vi "JV SNAKE AND LADDERS.vi"() -> ()   [LabVIEW 2018]
panel:
  out "String":string="PLAYER ONE TURN"
  out "Boolean":bool
  out "?":bool
  out "PLAYER 2 position":dbl
  out "PLAYER 1 position":dbl
  out "String 2":string="PLAYER TWO TURN"
  out "VALUE YOU GOT":dbl
  in  "stop":bool
  in  "THROW":bool
  out "Numeric":dbl
  out "DICE":u16(ring)
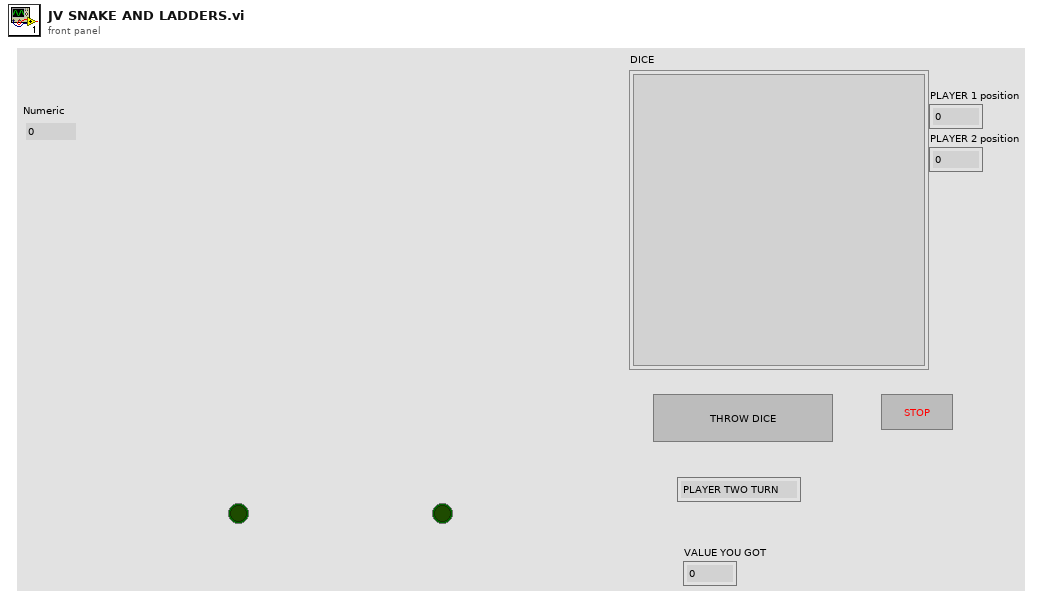
[diagram p1: front panel]
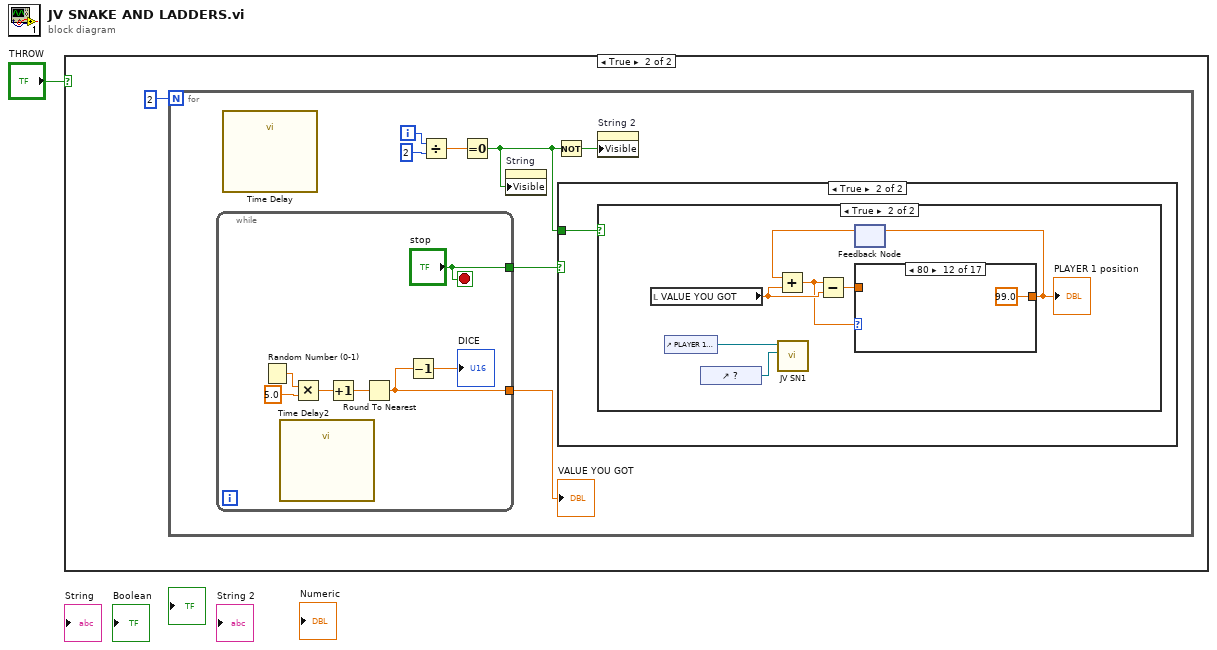
[diagram p0: block diagram]
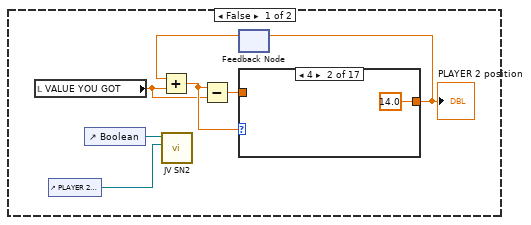
[diagram p4: hidden frame]
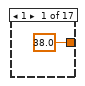
[diagram p5: hidden frame]
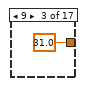
[diagram p6: hidden frame]
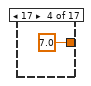
[diagram p7: hidden frame]
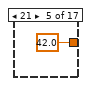
[diagram p8: hidden frame]
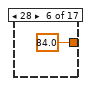
[diagram p9: hidden frame]
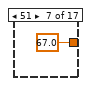
[diagram p10: hidden frame]
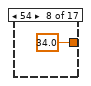
[diagram p11: hidden frame]
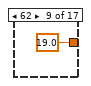
[diagram p12: hidden frame]
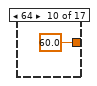
[diagram p13: hidden frame]
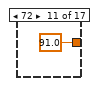
[diagram p14: hidden frame]
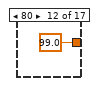
[diagram p15: hidden frame]
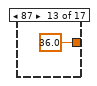
[diagram p16: hidden frame]
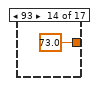
[diagram p17: hidden frame]
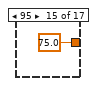
[diagram p18: hidden frame]
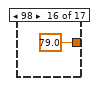
[diagram p19: hidden frame]
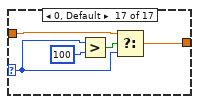
[diagram p20: hidden frame]
diagram:
  n1 = case shown="True" "THROW" {
    frame False {
    }
    frame True {
      n2 = for {
        N: 2 -> [_]
        i -> [w9]
        n3 = while {
          tunnel: [w69] -> w6
          tunnel: ["stop"] -> w5
          stop <- "stop" stop-if-true
          n4 = Random Number (0-1)() -> (number: 0 to 1=w73:dbl)
          n5 = call "Time Delay2"() -> ()  [unwired: 11 in, 1 out]
          n6 = Multiply(x=w73, y=5.0) -> (x*y=w71:dbl)
          n7 = Increment(x=w71) -> (x+1=w70:dbl)
          n8 = Round To Nearest(number=w70) -> (nearest integer value=w69:dbl)
          n9 = Decrement(x=w69) -> (x-1=→"DICE":dbl)
        }
        "VALUE YOU GOT" <- w6
        n10 = call "Time Delay"() -> ()  [unwired: 11 in, 1 out]
        n11 = Divide(x=w9, y=2) -> (x/y=w7:dbl)
        n12 = Equal To 0?(x=w7) -> (x = 0?=w3:bool)
        n13 = property on="String" class="Str"("Visible"=w3) -> ()  [unwired: 2 in, 2 out]
        n14 = Not(x=w3) -> (.not. x?=w4:bool)
        n15 = case shown="True" w5 {
          tunnel: w3 -> [_ w10]
          frame False {
          }
          frame True {
            n16 = case shown="True" w10 {
              frame False {
                n17 = local read "VALUE YOU GOT"() -> (w13:dbl)
                n18 = control-ref of="PLAYER 2 position"() -> (w11:refnum<vi>)
                n19 = control-ref of="Boolean"() -> (w12:refnum<vi>)
                n20 = call "JV SN2.vi"("reference"=w11, "Boolean in"=w12) -> ()  [unwired: 10 in]
                n21 = feedback #1() -> (w17:dbl)  [unwired: 1 in]
                n22 = Add(x=w17, y=w13) -> (x+y=w16:dbl)
                n23 = Subtract(x=w16, y=w13) -> (x-y=w15:dbl)
                n24 = case shown="4" w16 {
                  selector: w16 -> [_ _ _ _ _ _ _ _ _ _ _ _ _ _ _ _ w35]
                  tunnel: [38.0 ("f") 14.0 ("f") 31.0 ("f") 7.0 ("f") 42.0 ("f") 84.0 ("f") 67.0 ("f") 34.0 ("f") 19.0 ("f") 60.0 ("f") 91.0 ("f") 99.0 ("f") 36.0 ("f") 73.0 ("f") 75.0 ("f") 79.0 ("f") w37] -> w14
                  tunnel: w15 -> [_ _ _ _ _ _ _ _ _ _ _ _ _ _ _ _ w36]
                  frame 1 {
                  }
                  frame 4 {
                  }
                  frame 9 {
                  }
                  frame 17 {
                  }
                  frame 21 {
                  }
                  frame 28 {
                  }
                  frame 51 {
                  }
                  frame 54 {
                  }
                  frame 62 {
                  }
                  frame 64 {
                  }
                  frame 72 {
                  }
                  frame 80 {
                  }
                  frame 87 {
                  }
                  frame 93 {
                  }
                  frame 95 {
                  }
                  frame 98 {
                  }
                  frame 0, Default {
                    n25 = Greater?(x=w35, y=100 ("x")) -> (0:w38:bool)
                    n26 = Select(t=w36, s=w38, f=w35) -> (s? t:f=w37:dbl)
                  }
                }
                "PLAYER 2 position" <- w14
                n27 = feedback-in #1(w14) -> ()
              }
              frame True {
                n28 = local read "VALUE YOU GOT"() -> (w44:dbl)
                n29 = control-ref of="PLAYER 1 position"() -> (w40:refnum<vi>)
                n30 = control-ref of="?"() -> (w39:refnum<vi>)
                n31 = call "JV SN1.vi"("Bool Refnum"=w39, "Digital in"=w40) -> ()  [unwired: 10 in]
                n32 = feedback #2() -> (w45:dbl)  [unwired: 1 in]
                n33 = Add(x=w45, y=w44) -> (x+y=w42:dbl)
                n34 = Subtract(x=w42, y=w44) -> (x-y=w43:dbl)
                n35 = case shown="80" w42 {
                  selector: w42 -> [_ _ _ _ _ _ _ _ _ _ _ _ _ _ _ _ w63]
                  tunnel: [38.0 ("f") 14.0 ("f") 31.0 ("f") 7.0 ("f") 42.0 ("f") 84.0 ("f") 67.0 ("f") 34.0 ("f") 19.0 ("f") 60.0 ("f") 91.0 ("f") 99.0 ("f") 36.0 ("f") 73.0 ("f") 75.0 ("f") 79.0 ("f") w65] -> w41
                  tunnel: w43 -> [_ _ _ _ _ _ _ _ _ _ _ _ _ _ _ _ w64]
                  frame 1 {
                  }
                  frame 4 {
                  }
                  frame 9 {
                  }
                  frame 17 {
                  }
                  frame 21 {
                  }
                  frame 28 {
                  }
                  frame 51 {
                  }
                  frame 54 {
                  }
                  frame 62 {
                  }
                  frame 64 {
                  }
                  frame 72 {
                  }
                  frame 80 {
                  }
                  frame 87 {
                  }
                  frame 93 {
                  }
                  frame 95 {
                  }
                  frame 98 {
                  }
                  frame 0, Default {
                    n36 = Greater?(x=w63, y=100 ("x")) -> (0:w66:bool)
                    n37 = Select(t=w64, s=w66, f=w63) -> (s? t:f=w65:dbl)
                  }
                }
                "PLAYER 1 position" <- w41
                n38 = feedback-in #2(w41) -> ()
              }
            }
          }
        }
        n39 = property on="String 2" class="Str"("Visible"=w4) -> ()  [unwired: 2 in, 2 out]
      }
    }
  }
